vi "select_image_subtraction_value_of_SD_animal.vi"(9 "Image subtraction \nvalues of all animals":i32[](array[numeric])) -> (2 "Image subtraction \nvalue of SD animal":i32)   [LabVIEW 2011]
uses:
  Action Items.ctl
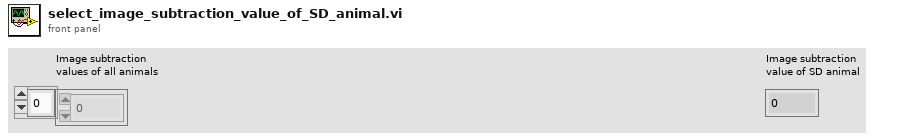
[diagram p1: front panel]
types:
  T1 = typedef "Action Items.ctl" = enum16{"Initialize", "Get"}
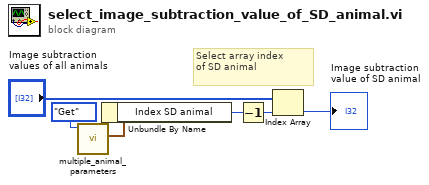
[diagram p0: block diagram]
diagram:
  # "Select array index\nof SD animal"
  n1 = call "multiple_animal_parameters.vi"("Action"=Action_Items."Get") -> ("Animal\nparameters"=w5:cluster{"# Animals":i32, "Index SD animal":i32})  [unwired: 10 in]
  n2 = Unbundle By Name(w5) -> ("Index SD animal"=w4:i32)
  n3 = Decrement(x=w4) -> (x-1=w3:i32)
  n4 = Index Array(array="Image subtraction \nvalues of all animals", index=w3) -> (element=→"Image subtraction \nvalue of SD animal":i32)
